vi "FlussdichteKorrektur.vi"(8 "error in":errorcluster, 11 "B-Array in":dbl[](array[numeric])) -> (0 "error out":errorcluster, 3 "B-Array out":dbl[](array[numeric]))   [LabVIEW 2016]
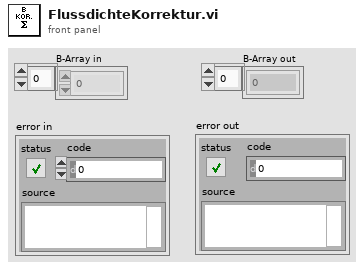
[diagram p1: front panel]
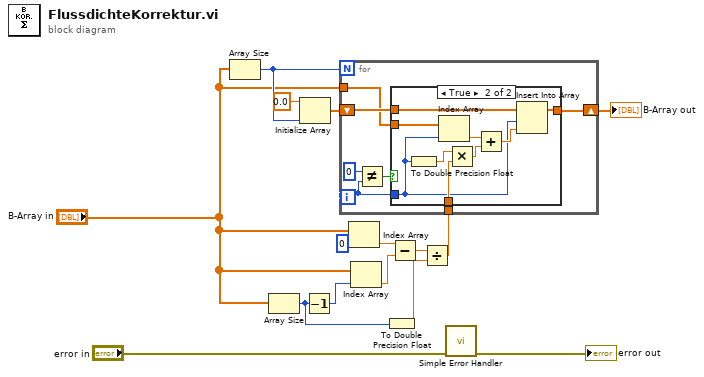
[diagram p0: block diagram]
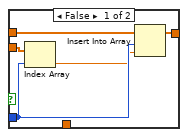
[diagram p2: hidden frame]
diagram:
  n1 = Array Size(array="B-Array in") -> (size(s)=w14:i32)
  n2 = Array Size(array="B-Array in") -> (size(s)=w10:i32)
  n3 = Initialize Array(0.0 ("element"), w14) -> (w12:dbl[])
  n4 = Decrement(x=w10) -> (x-1=w8:i32)
  n5 = Index Array(array="B-Array in", index=0) -> (element=w6:dbl)
  n6 = Index Array(array="B-Array in", index=w8) -> (element=w7:dbl)
  n7 = To Double Precision Float(number=w10) -> (double precision float=w11:dbl)
  n8 = Subtract(x=w6, y=w7) -> (x-y=w9:dbl)
  n9 = Divide(x=w9, y=w11) -> (x/y=w15:dbl)
  n10 = for {
    N: w14 -> [_]
    tunnel: "B-Array in" -> [w17]
    shift-right: [w18] -> w3
    shift-left: w12 -> [w19]
    tunnel: w15 -> [w16]
    i -> [w20]
    n11 = Not Equal?(x=0, y=w20) -> (x != y?=w21:bool)
    n12 = case shown="True" w21 {
      tunnel: w19 -> [w26 w36]
      tunnel: w20 -> [w24 w28]
      tunnel: [w27 w35] -> w18
      tunnel: w17 -> [w25 w34]
      tunnel: w16 -> [_ w30]
      frame False {
        n13 = Index Array(array=w25, index=w24) -> (element=w23:dbl)
        n14 = Insert Into Array(array=w26, index=w24, new element=w23) -> (w27:dbl[])
      }
      frame True {
        n15 = To Double Precision Float(number=w28) -> (double precision float=w31:dbl)
        n16 = Index Array(array=w34, index=w28) -> (element=w33:dbl)
        n17 = Multiply(x=w31, y=w30) -> (x*y=w32:dbl)
        n18 = Add(x=w33, y=w32) -> (x+y=w29:dbl)
        n19 = Insert Into Array(array=w36, index=w28, new element=w29) -> (w35:dbl[])
      }
    }
  }
  "B-Array out" <- w3
  n20 = call <vilib>:"Simple Error Handler.vi"("error in (no error)"="error in") -> ("error out"=→"error out":errorcluster)  [unwired: 4 in, 4 out]
